vi "Manual Correlation HPRF.vi"(5 "Ntheta":i32=16, 6 "Sensor Locations (cm)":dbl[][](array[numeric])=[[0.0, 0.0, -5.08], [11.43, 0.0, 0.0], [0.0, 11.43, 0.0], [-11.43, 0.0, 0.0], [0.0, -11.43, 0.0], [0.0, 0.0, 5.08]], 7 "Nr":i32=16, 8 "Sound Velocity (cm/s)":dbl=576000.0, 9 "Sampling Rate":i32=500000, 11 "Waveforms":dbl[][](array[numeric])) -> (2 "Coordinates (m)":cluster{"x":dbl, "y":dbl, "z":dbl})   [LabVIEW 2012]
uses:
  <vilib>/Analysis/2dsp.llb/1D Cross Correlation (DBL).vi
  <vilib>/Analysis/NI_AALPro.lvlib
panel:
  out "Signals":dbl[][](graph)
  out "output variable 3":dbl
  out "output variable 2":dbl
  out "output variable":dbl
  out "subarray 2":dbl[][](array[numeric])
  out "subarray":dbl[][](array[numeric])
  out "size(s)":i32[](array[numeric])
  out "theta":dbl
  out "r":dbl
  out "Correlation":dbl[][](graph)
  out "Lag Matrix":dbl[][](array[numeric])
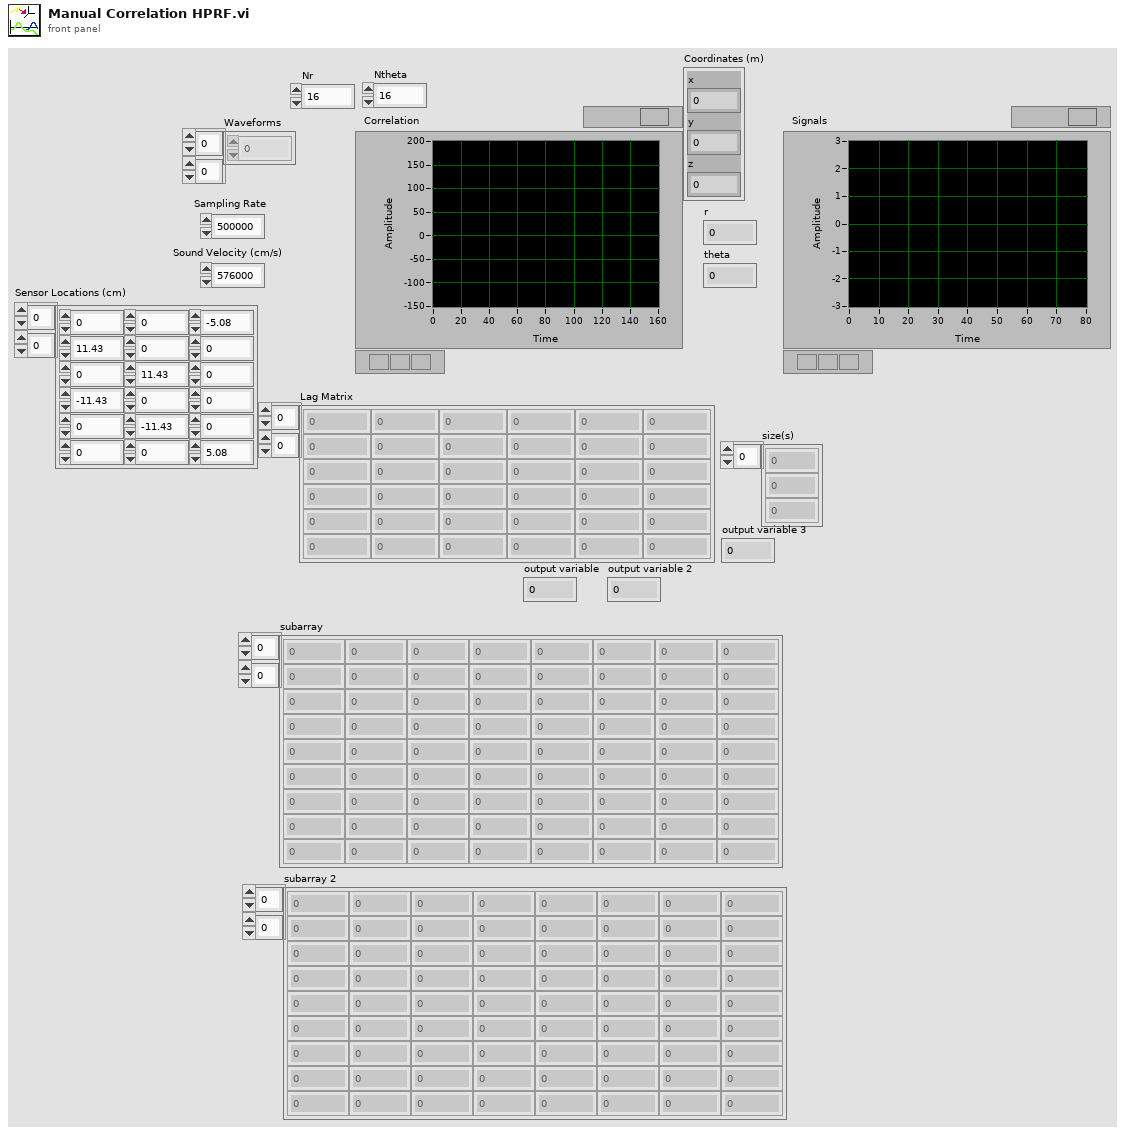
[diagram p1: front panel]
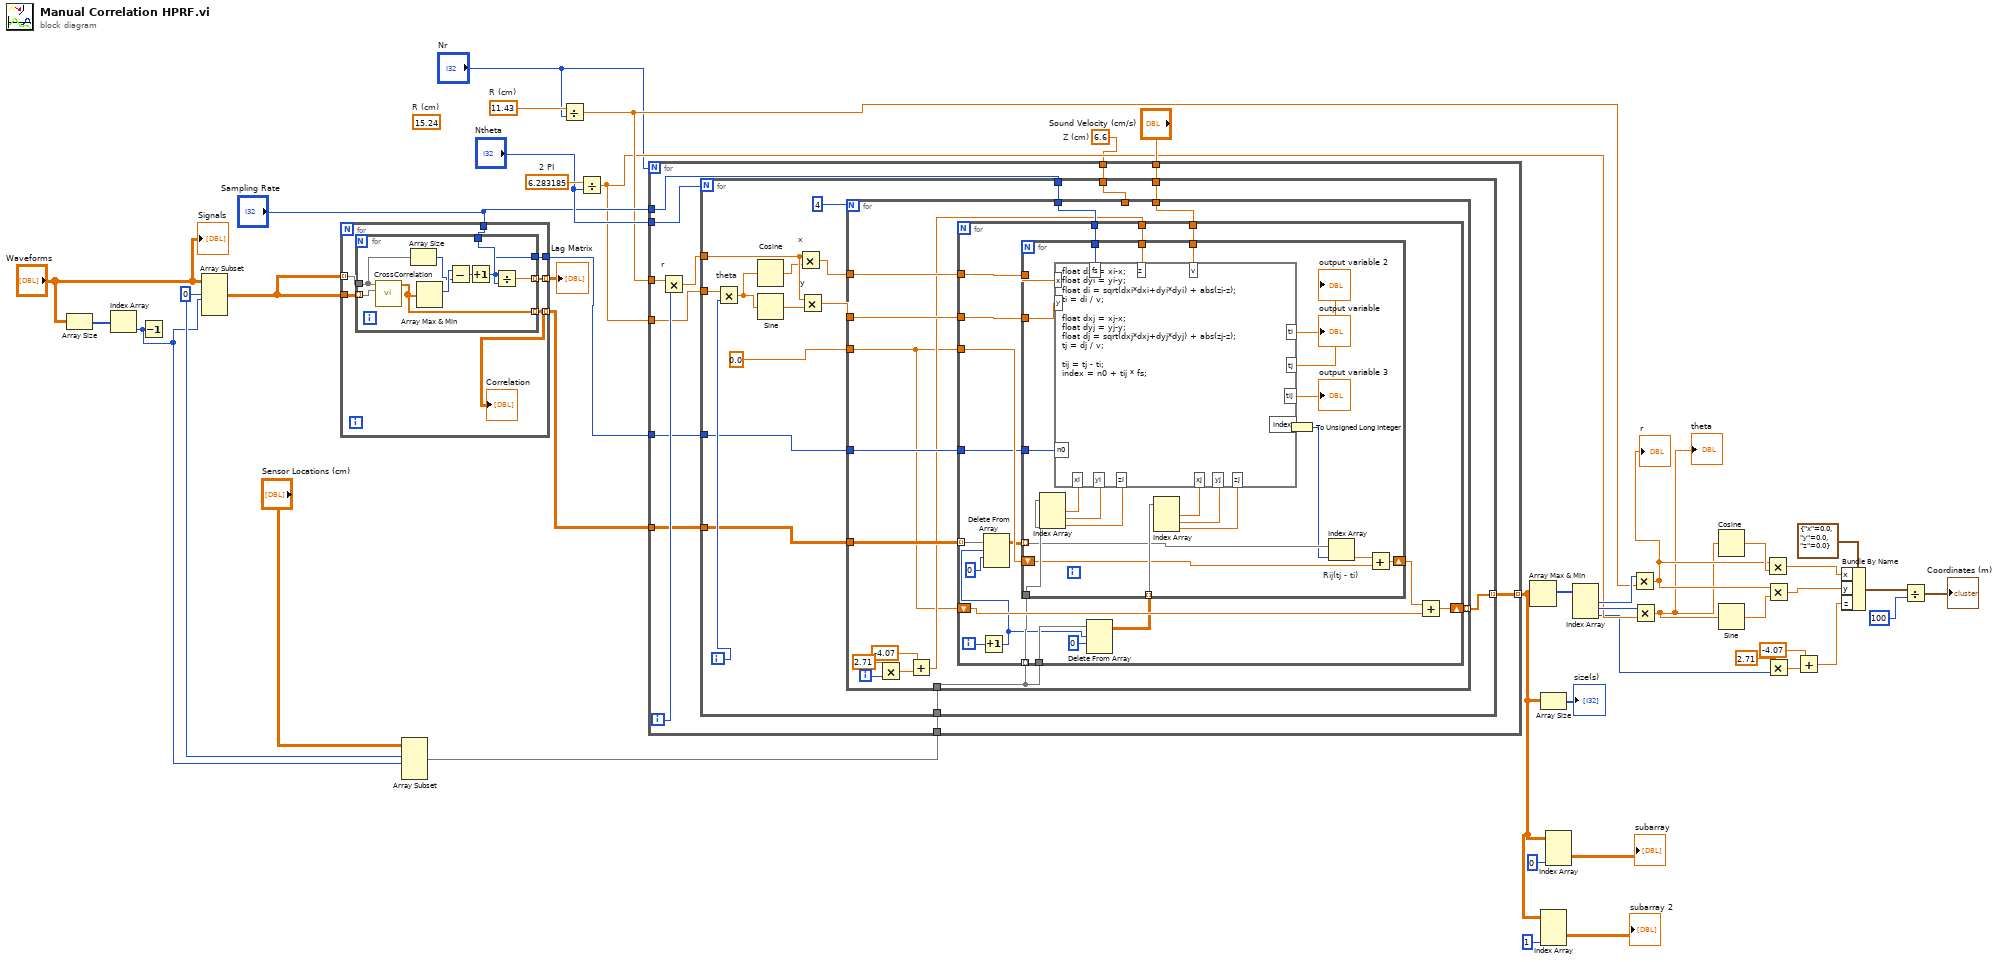
[diagram p0: block diagram]
diagram:
  (unwired) 15.24  # R (cm)
  w18 = 0 ("index")
  w42 = 11.43  # R (cm)
  w41 = 6.283185  # 2 PI
  w16 = 6.6  # Z (cm)
  n1 = Array Size(array="Waveforms") -> (size(s)=w3:i32[])
  n2 = Index Array(array=w3) -> (element=w1:i32)  [unwired: 1 in]
  n3 = Decrement(x=w1) -> ()  [unwired: 1 out]
  n4 = Array Subset(array="Waveforms", index (row)=w18, length (row)=w1) -> (w20:dbl[][])  [unwired: 2 in]
  n5 = for {
    tunnel: w20 -> [w48] mode=indexing
    tunnel: w20 -> [w49]
    tunnel: "Sampling Rate" -> [w47]
    tunnel: [w46] -> w43 mode=indexing
    tunnel: [w44] -> w36 mode=indexing
    tunnel: [w45] -> w37
    n6 = for {
      tunnel: w49 -> [w58] mode=indexing
      tunnel: w48 -> [w57]
      tunnel: w47 -> [w56]
      tunnel: [w55] -> w46 mode=indexing
      tunnel: [w52] -> w44 mode=indexing
      tunnel: [w53] -> w45
      n7 = call-poly <vilib>:"CrossCorrelation.vi"("Y"=w58, "X"=w57) -> ("Rxy"=w52:dbl[])  [unwired: 8 in, 1 out]
      n8 = Array Size(array=w57) -> (size(s)=w50:i32)
      n9 = Array Max & Min(array=w52) -> (max index (indices)=w51:i32)  [unwired: 3 out]
      n10 = Subtract(x=w51, y=w50) -> (x-y=w54:i32)
      n11 = Increment(x=w54) -> (x+1=w53:i32)
      n12 = Divide(x=w53, y=w56) -> (x/y=w55:dbl)
    }
    "Correlation" <- w44
  }
  "Lag Matrix" <- w43
  n13 = Array Subset(array="Sensor Locations (cm)", index (row)=w18, length (row)=w1) -> (w4:dbl[][])  [unwired: 2 in]
  n14 = Divide(x=w42, y="Nr") -> (x/y=w32:dbl)
  n15 = Divide(x=w41, y="Ntheta") -> (x/y=w31:dbl)
  n16 = for {
    N: "Nr" -> [_]
    tunnel: [w70] -> w5 mode=indexing
    tunnel: "Ntheta" -> [w69]
    tunnel: w32 -> [w68]
    tunnel: w31 -> [w66]
    tunnel: w4 -> [w65]
    tunnel: w16 -> [w64]
    tunnel: "Sound Velocity (cm/s)" -> [w63]
    tunnel: "Sampling Rate" -> [w62]
    tunnel: w37 -> [w61]
    tunnel: w36 -> [w60]
    i -> [w67]
    n17 = Multiply "r"(x=w68, y=w67) -> (x*y=w59:dbl)
    n18 = for {
      N: w69 -> [_]
      tunnel: [w86] -> w70 mode=indexing
      tunnel: w66 -> [w85]
      tunnel: w59 -> [w83]
      tunnel: w65 -> [w80]
      tunnel: w64 -> [w72]
      tunnel: w63 -> [w79]
      tunnel: w62 -> [w78]
      tunnel: w61 -> [w77]
      tunnel: w60 -> [w76]
      i -> [w84]
      n19 = Multiply "theta"(x=w85, y=w84) -> (x*y=w75:dbl)
      n20 = Cosine(x=w75) -> (cos(x)=w82:dbl)
      n21 = Sine(x=w75) -> (sin(x)=w81:dbl)
      n22 = Multiply "x"(x=w83, y=w82) -> (x*y=w74:dbl)
      n23 = Multiply "y"(x=w83, y=w81) -> (x*y=w73:dbl)
      n24 = for {
        N: 4 -> [_]
        tunnel: 0.0 -> [w88]
        tunnel: [w101] -> w86 mode=indexing
        tunnel: w80 -> [w100]
        tunnel: w79 -> [w99]
        tunnel: w78 -> [w98]
        tunnel: w77 -> [w97]
        tunnel: w76 -> [w96]
        tunnel: w74 -> [w95]
        tunnel: w73 -> [w94]
        tunnel: w72 -> [_]
        i -> [w93]
        n25 = Multiply(x=2.71, y=w93) -> (x*y=w91:dbl)
        n26 = Add(x=-4.07, y=w91) -> (x+y=w89:dbl)
        n27 = for {
          shift-right: [w117] -> w101
          shift-left: w88 -> [w118]
          tunnel: w88 -> [w120]
          tunnel: w95 -> [w116]
          tunnel: w94 -> [w115]
          tunnel: w100 -> [w114] mode=indexing
          tunnel: w100 -> [w108]
          tunnel: w89 -> [w113]
          tunnel: w99 -> [w112]
          tunnel: w98 -> [w111]
          tunnel: w97 -> [w110]
          tunnel: w96 -> [w105] mode=indexing
          i -> [w109]
          n28 = Increment(x=w109) -> (x+1=w102:i32)
          n29 = Delete From Array(array=w105, length=w102, index (row)=0) -> (array with subset deleted=w104:dbl[][])  [unwired: 1 in, 1 out]
          n30 = Delete From Array(array=w108, length=w102, index (row)=0) -> (array with subset deleted=w106:dbl[][])  [unwired: 1 in, 1 out]
          n31 = for {
            shift-right: [w128] -> w119
            shift-left: w120 -> [w126]
            tunnel: w116 -> [w139]
            tunnel: w115 -> [w138]
            tunnel: w106 -> [w142] mode=indexing
            tunnel: w114 -> [w143]
            tunnel: w113 -> [w141]
            tunnel: w112 -> [w140]
            tunnel: w111 -> [w133]
            tunnel: w110 -> [w132]
            tunnel: w104 -> [w130] mode=indexing
            n32 = Index Array(array=w143) -> (element #1=w137:dbl, element #2=w136:dbl, element #3=w125:dbl)  [unwired: 3 in]
            n33 = Index Array(array=w142) -> (element #1=w135:dbl, element #2=w134:dbl, element #3=w124:dbl)  [unwired: 3 in]
            n34 = formula code="float dxi = xi-x;\nfloat dyi = yi-y;\nfloat di = sqrt(dxi*dxi+dyi*dyi) + abs(zi-z);\nti = di / v;\n\nfloat dxj = xj-x;\nfloat dyj = yj-y;\nfloat dj = sqrt(dxj*dxj+dyj*dyj) + abs(zj-z);\ntj = dj / v;\n\ntij = tj - ti;\nindex = n0 + tij * fs;"("xi"=w137, "yi"=w136, "xj"=w135, "yj"=w134, "x"=w139, "y"=w138, "z"=w141, "v"=w140, "fs"=w133, "n0"=w132, "zi"=w125, "zj"=w124) -> ("index"=w131:dbl, "ti"=→"output variable":dbl, "tj"=→"output variable 2":dbl, "tij"=→"output variable 3":dbl)
            n35 = To Unsigned Long Integer(number=w131) -> (unsigned 32bit integer=w129:u32)
            n36 = Index Array "Rij(tj - ti)"(array=w130, index=w129) -> (element=w127:dbl)
            n37 = Add(x=w127, y=w126) -> (x+y=w128:dbl)
          }
          n38 = Add(x=w119, y=w118) -> (x+y=w117:dbl)
        }
      }
    }
  }
  n39 = Array Max & Min(array=w5) -> (max index (indices)=w35:i32[])  [unwired: 3 out]
  n40 = Array Size(array=w5) -> (size(s)=→"size(s)":i32[])
  n41 = Index Array(array=w5, index (dim 2)=1 ("disabled index (col)")) -> (element=→"subarray 2":dbl[][])  [unwired: 2 in]
  n42 = Index Array(array=w5, index (dim 2)=0 ("disabled index (col)")) -> (element=→"subarray":dbl[][])  [unwired: 2 in]
  n43 = Index Array(array=w35) -> (element #1=w34:i32, element #2=w33:i32, element #3=w12:i32)  [unwired: 3 in]
  n44 = Multiply(x=w34, y=w32) -> (x*y=w28:dbl)
  "r" <- w28
  n45 = Multiply(x=w33, y=w31) -> (x*y=w27:dbl)
  "theta" <- w27
  n46 = Cosine(x=w27) -> (cos(x)=w30:dbl)
  n47 = Sine(x=w27) -> (sin(x)=w29:dbl)
  n48 = Multiply ("x*y")(x=w28, y=w30) -> (x*y=w26:dbl)
  n49 = Multiply ("x*y")(x=w28, y=w29) -> (x*y=w25:dbl)
  n50 = Multiply(x=2.71, y=w12) -> (x*y=w14:dbl)
  n51 = Add(x=-4.07, y=w14) -> (x+y=w11:dbl)
  n52 = Bundle By Name(cluster=cluster{"x":dbl, "y":dbl, "z":dbl} {"x"=0.0, "y"=0.0, "z"=0.0} ("input cluster"), "x"=w26, "y"=w25, "z"=w11) -> (w23:cluster{"x":dbl, "y":dbl, "z":dbl})
  n53 = Divide(x=w23, y=100 ("index (row)")) -> (x/y=→"Coordinates (m)":cluster{"x":dbl, "y":dbl, "z":dbl})
  "Signals" <- "Waveforms"
